vi "Do.vi"(8 "error in (no error)":errorcluster, 10 "Actor in":refnum<class "Actor.lvclass">, 11 "CyclicMessage":refnum<class "MessageCycle.lvclass">) -> (0 "error out":errorcluster, 2 "Actor out":refnum<class "Actor.lvclass">)   [LabVIEW 2017, in "MessageCycle.lvclass"]
doc: "(<B>Filename</B>: Actor Framework.lvlib:Message.lvclass:Do.vi)\n\nDefines what a message does when it is received by an actor. Generally, a message instructs an actor to invoke one of its methods. By default, this method does nothing. A child class must override it to define behavior. Create a child class by using the Actor Framework Message Maker dialog box."
uses:
  <vilib>/gpm_packages/@cs/actor-framework-messages/Source/MessageCycle/MessageCycle.lvclass
  C:/Program Files/National Instruments/LabVIEW 2017/vi.lib/ActorFramework/Message/Message.lvclass
  <vilib>/ActorFramework/Actor/Actor.lvclass
  <vilib>/gpm_packages/@cs/actor-framework-messages/Source/MessageCycle/MessageCycle.lvclass/MessageCycle.ctl
  <vilib>/ActorFramework/Message Enqueuer/Message Enqueuer.lvclass/Message Enqueuer.ctl
  <vilib>/ActorFramework/Message Priority Queue/Priority Enqueue.vi
  <vilib>/ActorFramework/Message/Message.lvclass
  <vilib>/ActorFramework/Message Enqueuer/Message Enqueuer.lvclass
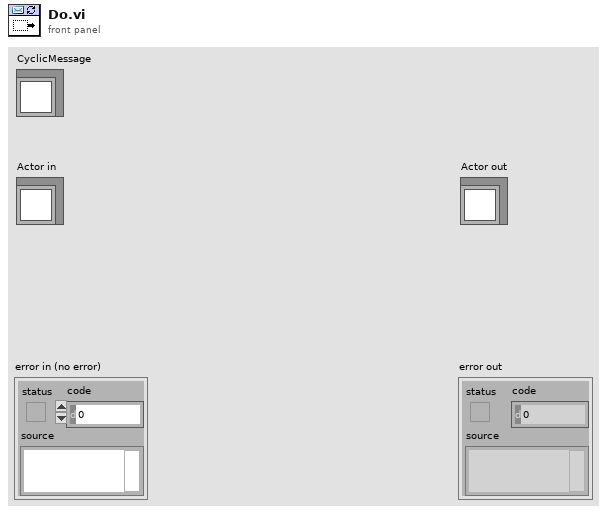
[diagram p1: front panel]
types:
  T1 = typedef "MessageCycle.lvclass/Message Cycle Notifications.ctl" = enum16{"Process Final Copy and Stop", "Stop Immediately", "Substitute Last Message and Stop"}
  T2 = typedef "Actor Framework.lvlib/Message Enqueuer.lvclass/Message Priority.ctl" = enum16{"Low", "Normal", "High"}
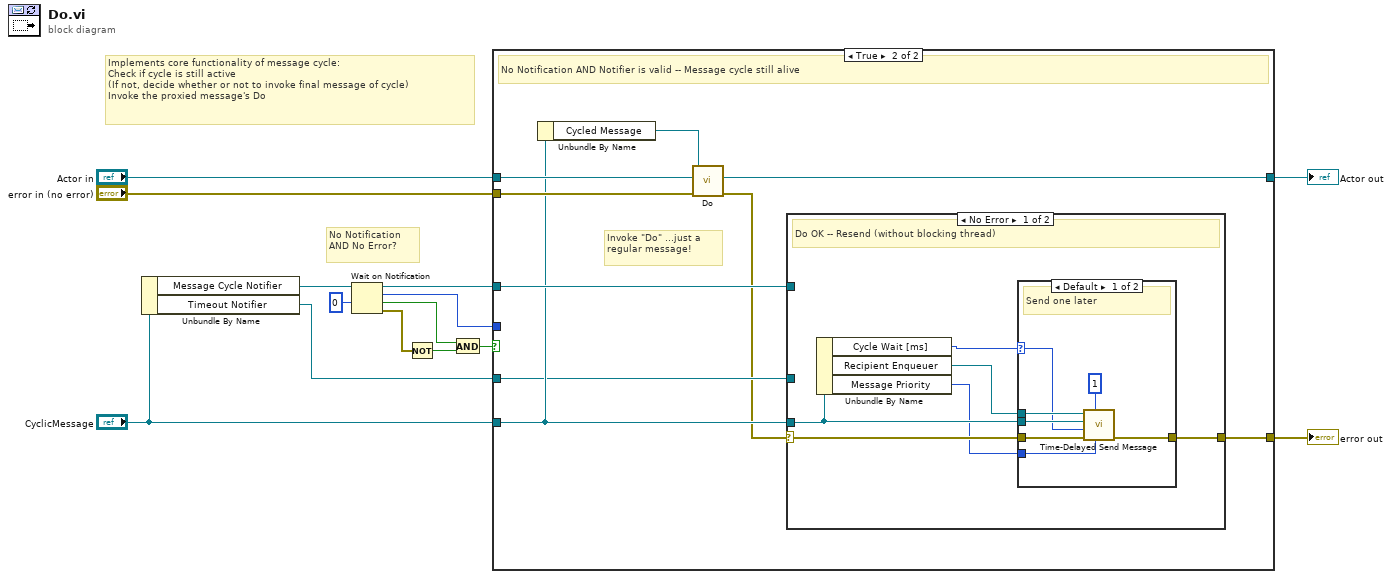
[diagram p0: block diagram]
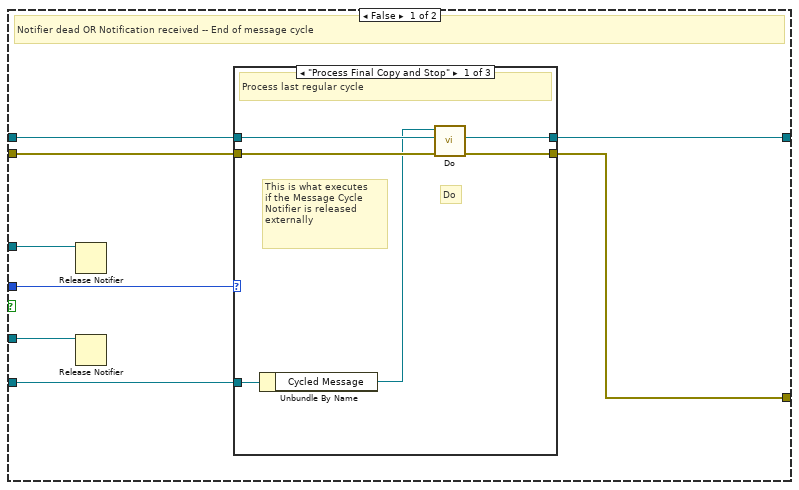
[diagram p2: hidden frame]
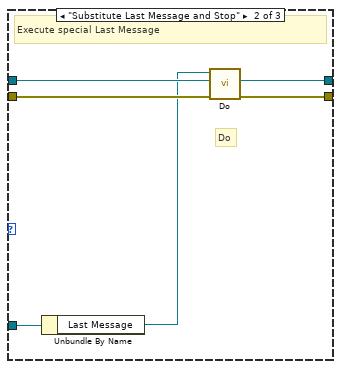
[diagram p3: hidden frame]
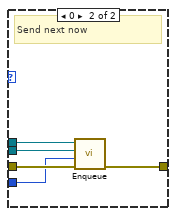
[diagram p5: hidden frame]
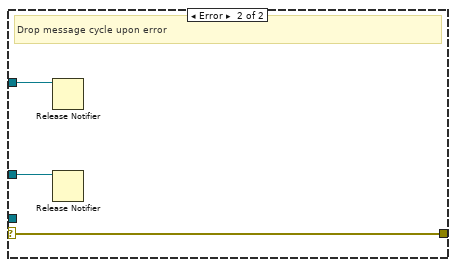
[diagram p6: hidden frame]
diagram:
  # "No Notification\nAND No Error?"
  # "Implements core functionality of message cycle:\nCheck if cycle is still active\n(If not, decide whether or not to invoke final message of cycle)\nInvoke the proxied message's Do"
  n1 = Unbundle By Name("CyclicMessage") -> ("Message Cycle Notifier"=w2:refnum<notifier>, "Timeout Notifier"=w1:refnum<notifier>)
  n2 = Wait on Notification(notifier=w2, timeout in ms (-1)=0) -> (notifier out=w9:refnum<notifier>, notification=w8:T1, timed out?=w6:bool, error out=w4:errorcluster)  [unwired: 2 in]
  n3 = Not(x=w4) -> (.not. x?=w5:bool)
  n4 = And(x=w6, y=w5) -> (x .and. y?=w7:bool)
  n5 = case shown="True" w7 {
    tunnel: [w21 w44] -> w13
    tunnel: "error in (no error)" -> [w18 w43]
    tunnel: "Actor in" -> [w22 w42]
    tunnel: [w17 w41] -> w12
    tunnel: w8 -> [w20 _]
    tunnel: w9 -> [w19 w45]
    tunnel: "CyclicMessage" -> [w16 w40]
    tunnel: w1 -> [w15 w38]
    frame False {
      # "Notifier dead OR Notification received -- End of message cycle"
      n6 = Release Notifier(notifier=w19) -> ()  [unwired: 2 in, 3 out]
      n7 = Release Notifier(notifier=w15) -> ()  [unwired: 2 in, 3 out]
      n8 = case shown="\"Process Final Copy and Stop\"" w20 {
        tunnel: w22 -> [w28 w34 w36]
        tunnel: [w27 w33 w36] -> w21
        tunnel: w18 -> [w26 w31 w35]
        tunnel: [w25 w32 w35] -> w17
        tunnel: w16 -> [w24 w30 _]
        frame "Process Final Copy and Stop" {
          # "This is what executes\nif the Message Cycle\nNotifier is released\nexternally"
          # "Do"
          # "Process last regular cycle"
          n9 = Unbundle By Name(w24) -> ("Cycled Message"=w23:refnum<class "Message.lvclass">)
          n10 = call-dynamic "Do.vi"("error in (no error)"=w26, "Actor in"=w28, "Message"=w23) -> ("error out"=w25:errorcluster, "Actor out"=w27:refnum<class "Actor.lvclass">)  [unwired: 7 in]
        }
        frame "Substitute Last Message and Stop" {
          # "Do"
          # "Execute special Last Message"
          n11 = Unbundle By Name(w30) -> ("Last Message"=w29:refnum<class "Message.lvclass">)
          n12 = call-dynamic "Do.vi"("error in (no error)"=w31, "Actor in"=w34, "Message"=w29) -> ("error out"=w32:errorcluster, "Actor out"=w33:refnum<class "Actor.lvclass">)  [unwired: 7 in]
        }
        frame "Stop Immediately" {
          # "No more!"
        }
      }
    }
    frame True {
      # "Invoke \"Do\" ...just a\nregular message!"
      # "No Notification AND Notifier is valid -- Message cycle still alive"
      n13 = Unbundle By Name(w40) -> ("Cycled Message"=w39:refnum<class "Message.lvclass">)
      n14 = call-dynamic "Do.vi"("error in (no error)"=w43, "Actor in"=w42, "Message"=w39) -> ("error out"=w37:errorcluster, "Actor out"=w44:refnum<class "Actor.lvclass">)  [unwired: 7 in]
      n15 = case shown="No Error" w37 {
        selector: w37 -> [w51 w66]
        tunnel: [w50 w66] -> w41
        tunnel: w40 -> [w48 _]
        tunnel: w45 -> [_ w65]
        tunnel: w38 -> [_ w64]
        frame No Error {
          # "Do OK -- Resend (without blocking thread)"
          n16 = Unbundle By Name(w48) -> ("Cycle Wait [ms]"=w46:i32, "Recipient Enqueuer"=w49:refnum<class "Message Enqueuer.lvclass">, "Message Priority"=w47:T2)
          n17 = case shown="Default" w46 {
            selector: w46 -> [w53 _]
            tunnel: w51 -> [w58 w63]
            tunnel: [w57 w62] -> w50
            tunnel: w49 -> [w56 w61]
            tunnel: w48 -> [w55 w60]
            tunnel: w47 -> [w54 w59]
            frame Default {
              # "Send one later"
              n18 = call <vilib>:"Time-Delayed Send Message.vi"("Message Priority (Normal)"=w54, "# Copies (0 = infinite repeat)"=u32 1, "error in (no error)"=w58, "Milliseconds To Wait"=w53, "Message"=w55, "Message Enqueuer"=w56) -> ("error out"=w57:errorcluster)  [unwired: 4 in, 1 out]
            }
            frame 0 {
              # "Send next now"
              n19 = call <vilib>:"Enqueue.vi"("error in (no error)"=w63, "Message Priority (Normal)"=w59, "Message"=w60, "Message Enqueuer in"=w61) -> ("error out"=w62:errorcluster)  [unwired: 6 in, 1 out]
            }
          }
        }
        frame Error {
          # "Drop message cycle upon error"
          n20 = Release Notifier(notifier=w65) -> ()  [unwired: 2 in, 3 out]
          n21 = Release Notifier(notifier=w64) -> ()  [unwired: 2 in, 3 out]
        }
      }
    }
  }
  "error out" <- w12
  "Actor out" <- w13
